vi "Byte Buffer.Read (String).vi"(8 "error in (no error)":errorcluster, 9 "size":i64, 10 "buffer offset":u64, 11 "Byte Buffer in":refnum<class "Byte Buffer.lvclass">) -> (0 "error out":errorcluster, 1 "string":string, 2 "new buffer offset":u64, 3 "Byte Buffer out":refnum<class "Byte Buffer.lvclass">)   [LabVIEW 2016, in "VeriStand Data.lvlib" / "Byte Buffer.lvclass"]
doc: "Reads <B>count</B> elements of data from the provided <B>Byte Buffer</B> at location <B>buffer offset</B> in the format of the data type specified."
uses:
  Byte Buffer.lvclass
  Byte Buffer.lvclass/Byte Buffer.ctl
  Byte Buffer.Get Buffer Pointer.vi
  Byte Buffer.Get Buffer Size.vi
  Memory Management/Memory Management.MoveByteBlock.Write (String).vi
  Memory Management/Memory Management.Handle Return.vi
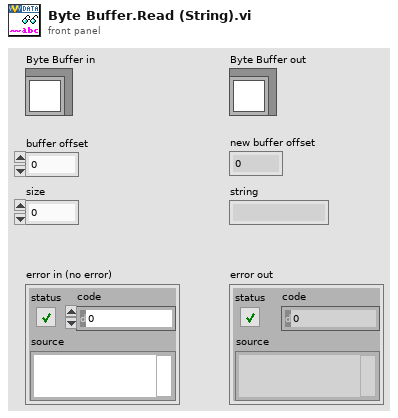
[diagram p1: front panel]
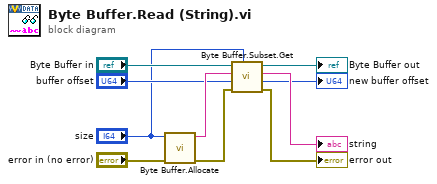
[diagram p0: block diagram]
diagram:
  n1 = call "Byte Buffer.Allocate.vi"("error in (no error)"="error in (no error)", "size"="size") -> ("error out"=w10:errorcluster, "buffer"=w4:string)  [unwired: 8 in]
  n2 = call "Byte Buffer.Subset.Get.vi"("length (-1: rest)"="size", "error in (no error)"=w10, "offset (0)"="buffer offset", "allocated string in"=w4, "Byte Buffer in"="Byte Buffer in") -> ("error out"=→"error out":errorcluster, "new buffer offset"=→"new buffer offset":u64, "string out"=→"string":string, "Byte Buffer out"=→"Byte Buffer out":refnum<class "Byte Buffer.lvclass">)  [unwired: 3 in]
